vi "Get Menu Items.vi"(8 "error in":errorcluster, 9 "GUID":string, 10 "Item Ref":T1 format="%.0x", 11 "System Explorer Dispatcher in":refnum<class "System Explorer Dispatcher.lvclass">) -> (0 "error out":errorcluster, 2 "Menu Items":cluster{"Name":string, "Enabled?":bool}[](array[cluster]), 3 "System Explorer Dispatcher out":refnum<class "System Explorer Dispatcher.lvclass">)   [LabVIEW 2020, in "Ballard MIL-STD-1553 System Explorer.lvlib" / "Implementation.lvlib" / "System Explorer Dispatcher.lvclass"]
uses:
  System Explorer Dispatcher.lvclass
  <vilib>/NI VeriStand/Custom Device API/Custom Device Item Ref.ctl
  Scripting/Constants.vi
  Scripting/Ballard MIL-STD-1553 Scripting.lvlib
  <vilib>/NI VeriStand/Custom Device API/Custom Device API.lvlib
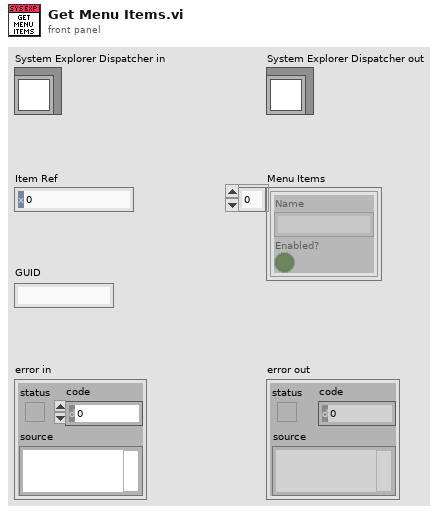
[diagram p1: front panel]
types:
  T1 = typedef "Custom Device API.lvlib/Custom Device Item Ref.ctl" = u64
  T2 = map{string, cluster{"Name":string, "Enabled?":bool}[]}
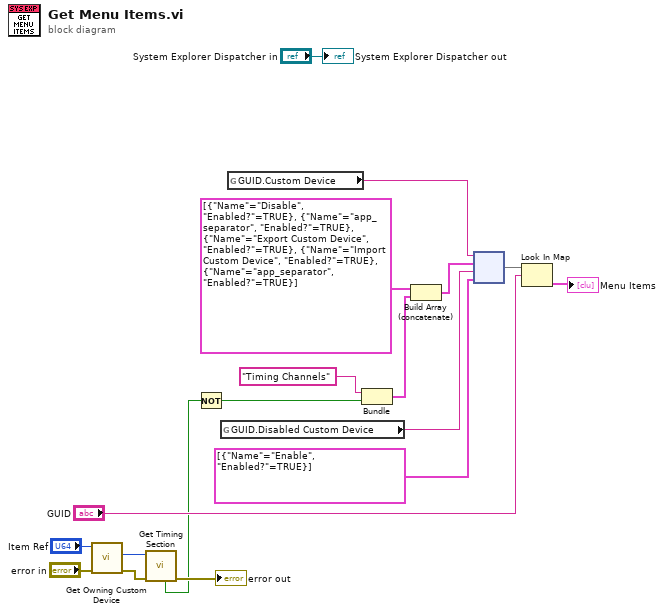
[diagram p0: block diagram]
diagram:
  n1 = call "Get Owning Custom Device.vi"("error in"="error in", "item"="Item Ref") -> ("error out"=w2:errorcluster, "owning custom device"=w1:T1)  [unwired: 7 in, 1 out]
  n2 = call "Get Timing Section.vi"("error in"=w2, "custom device in"=w1) -> ("error out"=→"error out":errorcluster, "found"=w9:bool)  [unwired: 6 in, 2 out]
  n3 = Not(x=w9) -> (.not. x?=w5:bool)
  n4 = global read "Constants.vi" "GUID.Disabled Custom Device"() -> (w3:string)
  n5 = global read "Constants.vi" "GUID.Custom Device"() -> (w4:string)
  n6 = Bundle("Name"="Timing Channels", w5) -> (w8:cluster{"Name":string, bool})  [unwired: 1 in]
  n7 = Build Array (concatenate)(cluster{"Name":string, "Enabled?":bool}[] [{"Name"="Disable", "Enabled?"=TRUE}, {"Name"="app_separator", "Enabled?"=TRUE}, {"Name"="Export Custom Device", "Enabled?"=TRUE}, {"Name"="Import Custom Device", "Enabled?"=TRUE}, {"Name"="app_separator", "Enabled?"=TRUE}] ("Menu Items"), w8) -> (w6:cluster{"Name":string, "Enabled?":bool}[])
  n8 = node(w4, w6, w3, cluster{"Name":string, "Enabled?":bool}[] [{"Name"="Enable", "Enabled?"=TRUE}] ("Menu Items")) -> (w17:T2)
  n9 = Look In Map(map=w17, key="GUID") -> (value=→"Menu Items":cluster{"Name":string, "Enabled?":bool}[])  [unwired: 1 in, 1 out]
  "System Explorer Dispatcher out" <- "System Explorer Dispatcher in"
